vi "Linear Scaling with Points.vi"(7 "x":dbl, 12 "Point1":cluster{"x1":dbl, "y1":dbl}, 13 "Point2":cluster{"x2":dbl, "y2":dbl}) -> (8 "y":dbl)   [LabVIEW 2018]
panel:
  # "y=ax+b"
  # "This is just an example - you should create your own scaling!"
  # "Hans-Petter Halvorsen\nhans.p.halvorsen@hit.no\nTelemark University College \nDepartment of Electrical Engineering, Information Technology and Cybernetics"
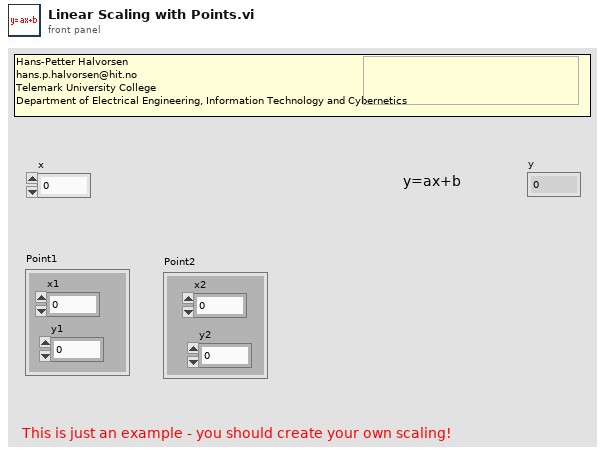
[diagram p1: front panel]
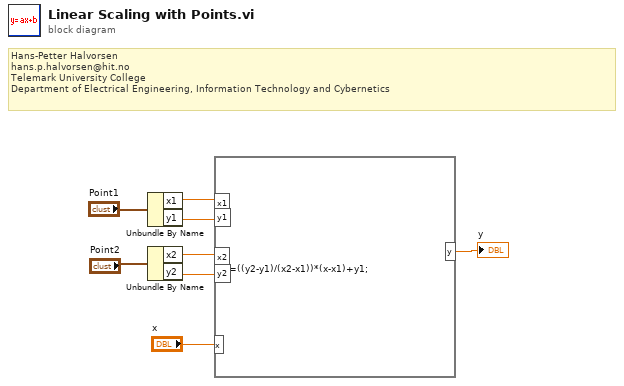
[diagram p0: block diagram]
diagram:
  # "Hans-Petter Halvorsen\nhans.p.halvorsen@hit.no\nTelemark University College \nDepartment of Electrical Engineering, Information Technology and Cybernetics"
  n1 = Unbundle By Name("Point1") -> ("x1"=w4:dbl, "y1"=w3:dbl)
  n2 = Unbundle By Name("Point2") -> ("x2"=w2:dbl, "y2"=w1:dbl)
  n3 = formula code="y=((y2-y1)/(x2-x1))*(x-x1)+y1;"("x1"=w4, "y1"=w3, "x2"=w2, "y2"=w1, "x"="x") -> ("y"=→"y":dbl)
